vi "CSGaussmeter.init.vi"(0 "i ref in":refnum<vi>, 11 "error in":errorcluster) -> (4 "i ref out":refnum<vi>, 15 "error out":errorcluster)   [LabVIEW 2014, in "CSGaussmeter.lvlib"]
doc: "Dieses VI liest alle Parameter aus dem Gerät aus\n\nThis VI reads all parameters from the device"
uses:
  CSGaussmeter.lvlib
  instr.lib/FH_55/TypeDef/Temp_Unit.ctl
  CS_Core/CSObj/CSObj.lvlib
  CSlibraries/UtilityLib/UtilityLib.lvlib
  CS_Core/CSApplicationBaseClasses/DeviceBase/DeviceBase.lvlib
  instr.lib/FH_55/FH 55.lvlib
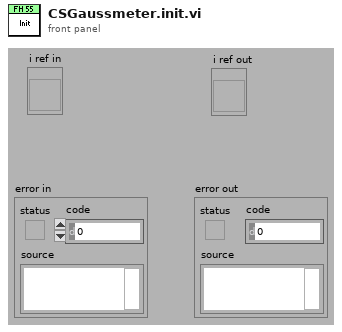
[diagram p1: front panel]
types:
  T1 = typedef "FH 55.lvlib/Temp_Unit.ctl" = enum16{"Temp off", "Celsius", "Fahrenheit"}
  T2 = typedef "CSGaussmeter.lvlib/CSGaussmeter.i attribute.ctl" = cluster{"Name":string, "VISA Resource Name":refnum<visa-resource-name>, "actValues":cluster{" Limit":bool, "Unit ":T3, "Temp_Unit":T1, "Max":T4, " Filter":bool, " Peak":bool, " Auto_Range":bool, "Range":T5, " Rel":bool, " CTemp":bool, " CField":bool, "AC_DC ":bool, "Set_lower":cluster{"Numeric":dbl, "Cancel Button":bool, "Unit":T6}, "Set_upper":cluster{"Numeric":dbl, "Cancel Button":bool, "Unit":T6}, "Set_Rel":cluster{"Numeric":dbl, "Cancel Button":bool, "Unit":T6}, "Zero":bool, " Local":bool, "Reset":bool, " Init":bool}, "FH 55 Gauss-/Teslameter":T7, "MAX_Value":T8, "MIN_Value":T8, "Rel_Value":T8, "Array ":string[], "LIMU":dbl, " LIML":dbl, "Messwerte 2":string, "Messwerte ":cluster{"Numeric":i32, "OK Button":bool}, "serviceID":cluster{"Current ID":i32, "Unit ID":i32, "Temp ID":i32, "Name ID \n":i32, "Visa ID ":i32}, "setValues ":cluster{" Limit":bool, "Unit ":T3, "Temp_Unit":T1, "Max":T4, " Filter":bool, " Peak":bool, " Auto_Range":bool, "Range":T5, " Rel":bool, " CTemp":bool, " CField":bool, "AC_DC ":bool, "Set_lower":cluster{"Numeric":dbl, "Cancel Button":bool, "Unit":T6}, "Set_upper":cluster{"Numeric":dbl, "Cancel Button":bool, "Unit":T6}, "Set_Rel":cluster{"Numeric":dbl, "Cancel Button":bool, "Unit":T6}, "Zero":bool, " Local":bool, "Reset":bool, " Init":bool}}
  T3 = typedef "FH 55.lvlib/Unit.ctl" = enum16{"T", "G", "A/m"}
  T4 = typedef "FH 55.lvlib/Max.ctl" = enum16{"MAX off", "Show MAX", "MAX/MIN"}
  T5 = typedef "FH 55.lvlib/Range.ctl" = enum16{"1", "2", "3", "4", "5", "6", "7"}
  T6 = typedef "FH 55.lvlib/Unit2.ctl" = enum16{"mT", "G", "kA/m"}
  T7 = typedef "FH 55.lvlib/Display.ctl" = cluster{"current value":string, "Limit":string, "Remote":string, "function ":string, "Cluster":cluster{"AC/DC":string, "Auto":string, "Filter":string, "Range":string, "Rel":string, "Peak":string}}
  T8 = typedef "FH 55.lvlib/Value_String.ctl" = cluster{"Numeric":dbl, "String":string}
  T9 = cluster{"VISA Resource Name":refnum<visa-resource-name>}
  T10 = typedef "FH 55.lvlib/VisaCluster.ctl" = cluster{"VISA Resource Name":refnum<visa-resource-name>}
  T11 = cluster{"Numeric":dbl, "Cancel Button":bool, "Unit":T6}
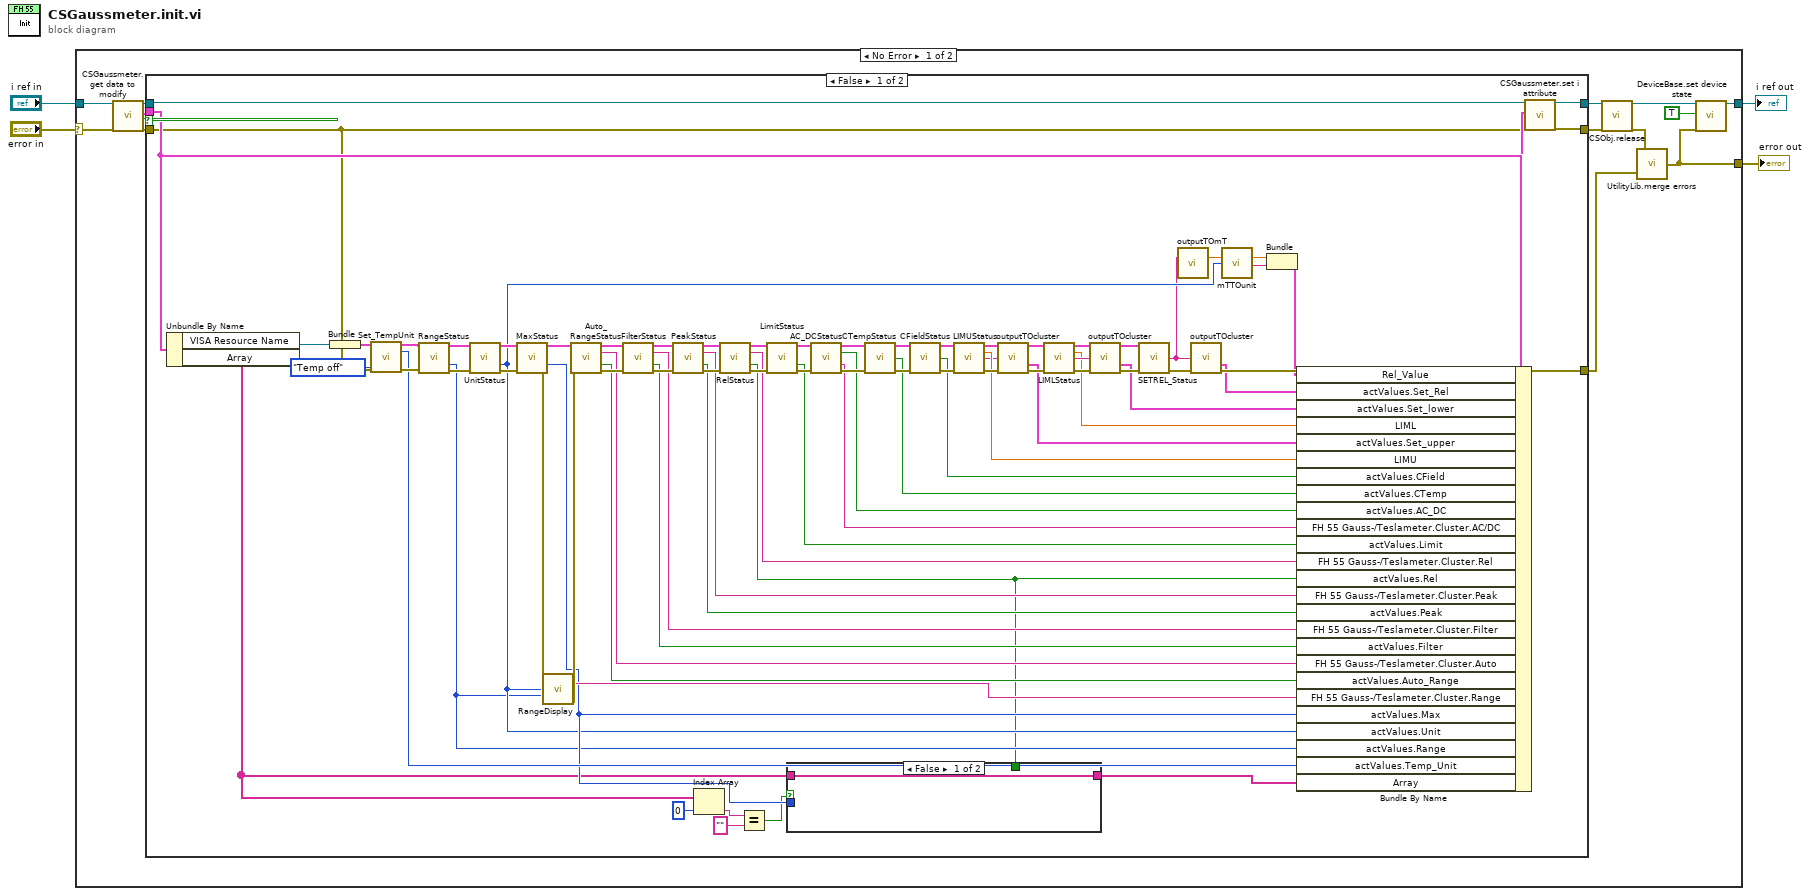
[diagram p0: block diagram]
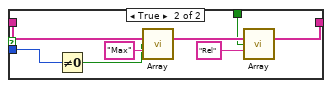
[diagram p2: hidden frame]
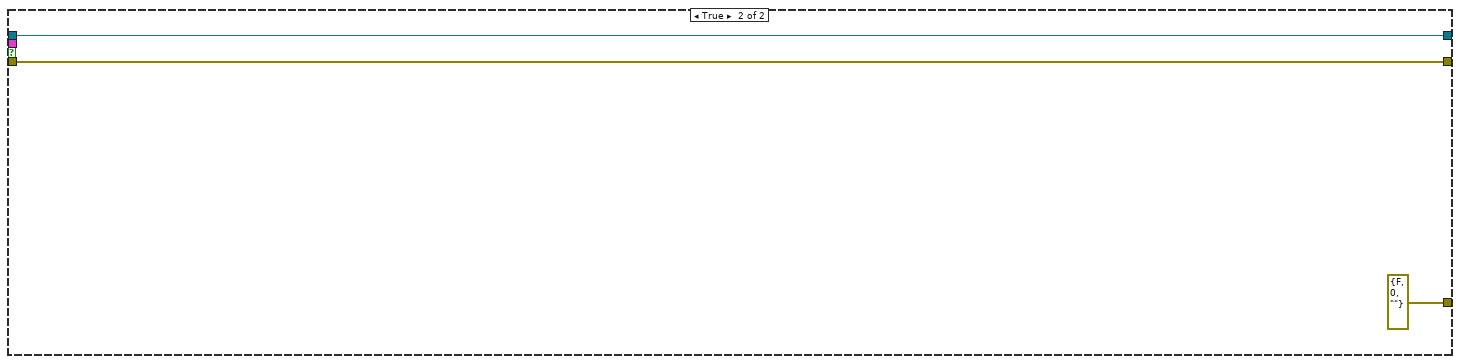
[diagram p3: hidden frame]
diagram:
  n1 = case shown="No Error" "error in" {
    selector: "error in" -> [w9 w109]
    tunnel: "i ref in" -> [w10 w110]
    tunnel: [w12 w110] -> w2
    tunnel: [w11 w109] -> w1
    frame No Error {
      n2 = call "CSGaussmeter.get data to modify.vi"("i ref in"=w10, "error in (no error)"=w9) -> ("i ref out"=w5:refnum<vi>, "i attribute"=w6:T2, "timed out"=w7:bool, "error out"=w8:errorcluster)  [unwired: 14 in]
      n3 = case shown="False" w7 {
        tunnel: w5 -> [w58 w106]
        tunnel: w8 -> [w55 w108]
        tunnel: w6 -> [w63 _]
        tunnel: [w57 w108] -> w17
        tunnel: [w53 errorcluster {"status"=FALSE, "code"=0, "source"=""} ("error out")] -> w18
        tunnel: [w59 w106] -> w15
        frame False {
          n4 = Unbundle By Name(w63) -> ("VISA Resource Name"=w96:refnum<visa-resource-name>, "Array"=w32:string[])
          n5 = Bundle("VISA Resource Name"=w96) -> (w60:T9)  [unwired: 1 in]
          n6 = call "Set_TempUnit.vi"("VisaCluster"=w60, "Temp_Unit"=Temp_Unit."Temp off", "error in (no error)"=w55) -> ("VisaCluster"=w72:T10, "Temp_Unit"=w46:T1, "error out"=w71:errorcluster)  [unwired: 9 in, 1 out]
          n7 = call "RangeStatus.vi"("VisaCluster"=w72, "error in (no error)"=w71) -> ("VisaCluster"=w80:T10, "Range"=w34:T5, "error out"=w78:errorcluster)  [unwired: 10 in, 1 out]
          n8 = call "UnitStatus.vi"("VisaCluster"=w80, "error in (no error)"=w78) -> ("VisaCluster"=w79:T10, "Unit"=w35:T3, "error out"=w77:errorcluster)  [unwired: 10 in, 1 out]
          n9 = call "MaxStatus.vi"("VisaCluster"=w79, "error in (no error)"=w77) -> ("VisaCluster"=w85:T10, "Max"=w36:T4, "error out"=w70:errorcluster)  [unwired: 10 in, 1 out]
          n10 = call "RangeDisplay.vi"("Unit"=w35, "Range"=w34, "error in (no error)"=w70) -> ("Display"=w37:string, "error out"=w69:errorcluster)  [unwired: 10 in, 1 out]
          n11 = call "Auto_RangeStatus.vi"("VisaCluster"=w85, "error in (no error)"=w69) -> ("VisaCluster"=w95:T10, "Display"=w39:string, "Auto_Range"=w38:bool, "error out"=w90:errorcluster)  [unwired: 9 in, 1 out]
          n12 = call "FilterStatus.vi"("VisaCluster"=w95, "error in (no error)"=w90) -> ("VisaCluster"=w94:T10, "Display"=w41:string, "Filter"=w40:bool, "error out"=w89:errorcluster)  [unwired: 9 in, 1 out]
          n13 = call "PeakStatus.vi"("VisaCluster"=w94, "error in (no error)"=w89) -> ("VisaCluster"=w93:T10, "Display"=w43:string, "Peak"=w42:bool, "error out"=w88:errorcluster)  [unwired: 9 in, 1 out]
          n14 = Index Array(array=w32, index=0) -> (element=w30:string)
          n15 = call "RelStatus.vi"("VisaCluster"=w93, "error in (no error)"=w88) -> ("VisaCluster"=w92:T10, "Display"=w44:string, "Rel"=w33:bool, "error out"=w87:errorcluster)  [unwired: 9 in, 1 out]
          n16 = Equal?(x=w30, y="") -> (x = y?=w28:bool)
          n17 = call "LimitStatus.vi"("VisaCluster"=w92, "error in (no error)"=w87) -> ("VisaCluster"=w91:T10, "Limit"=w45:bool, "error out"=w86:errorcluster)  [unwired: 10 in, 1 out]
          n18 = case shown="False" w28 {
            tunnel: [w97 w101] -> w51
            tunnel: w36 -> [_ w100]
            tunnel: w33 -> [_ w99]
            tunnel: w32 -> [w97 w98]
            frame False {
            }
            frame True {
              n19 = Not Equal To 0?(x=w100) -> (x != 0?=w102:bool)
              n20 = call "Array.vi"("Array"=w98, "Boolean"=w102, "String"="Max") -> ("Array"=w103:string[])  [unwired: 12 in]
              n21 = call "Array.vi"("Array"=w103, "Boolean"=w99, "String"="Rel") -> ("Array"=w101:string[])  [unwired: 12 in]
            }
          }
          n22 = call "AC_DCStatus.vi"("VisaCluster"=w91, "error in (no error)"=w86) -> ("VisaCluster"=w84:T10, "AC_DC"=w20:bool, "Display"=w19:string, "error out"=w82:errorcluster)  [unwired: 9 in, 1 out]
          n23 = call "CTempStatus.vi"("VisaCluster"=w84, "error in (no error)"=w82) -> ("VisaCluster"=w83:T10, "CTemp"=w22:bool, "error out"=w81:errorcluster)  [unwired: 10 in, 1 out]
          n24 = call "CFieldStatus.vi"("VisaCluster"=w83, "error in (no error)"=w81) -> ("VisaCluster"=w75:T10, "CField"=w21:bool, "error out"=w76:errorcluster)  [unwired: 10 in, 1 out]
          n25 = call "LIMUStatus.vi"("VisaCluster"=w75, "error in (no error)"=w76) -> ("VisaCluster"=w74:T10, "Numeric"=w27:dbl, "Message Out"=w26:string, "error out"=w68:errorcluster)  [unwired: 10 in]
          n26 = call "outputTOcluster.vi"("Input"=w26, "error in (no error)"=w68) -> ("Set_lower"=w47:T11, "error out"=w67:errorcluster)  [unwired: 11 in, 1 out]
          n27 = call "LIMLStatus.vi"("VisaCluster"=w74, "error in (no error)"=w67) -> ("VisaCluster"=w73:T10, "Numeric"=w24:dbl, "Message Out"=w25:string, "error out"=w66:errorcluster)  [unwired: 10 in]
          n28 = call "outputTOcluster.vi"("Input"=w25, "error in (no error)"=w66) -> ("Set_lower"=w48:T11, "error out"=w65:errorcluster)  [unwired: 11 in, 1 out]
          n29 = call "SETREL_Status.vi"("VisaCluster"=w73, "error in (no error)"=w65) -> ("Answer"=w23:string, "error out"=w54:errorcluster)  [unwired: 10 in, 2 out]
          n30 = call "outputTOmT.vi"("Input"=w23) -> ("Numeric"=w64:dbl)  [unwired: 13 in, 1 out]
          n31 = call "outputTOcluster.vi"("Input"=w23, "error in (no error)"=w54) -> ("Set_lower"=w49:T11, "error out"=w53:errorcluster)  [unwired: 11 in, 1 out]
          n32 = call "mTTOunit.vi"("Numeric"=w64, "Unit"=w35) -> ("Numeric 2"=w62:dbl, "Display"=w61:string)  [unwired: 11 in, 1 out]
          n33 = Bundle("Numeric 2"=w62, "Display"=w61) -> (w50:cluster{"Numeric 2":dbl, "Display":string})  [unwired: 1 in]
          n34 = Bundle By Name(cluster=w63, "Rel_Value"=w50, "actValues.Set_Rel"=w49, "actValues.Set_lower"=w48, "LIML"=w24, "actValues.Set_upper"=w47, "LIMU"=w27, "actValues.CField"=w21, "actValues.CTemp"=w22, "actValues.AC_DC"=w20, "FH 55 Gauss-/Teslameter.Cluster.AC/DC"=w19, "actValues.Limit"=w45, "FH 55 Gauss-/Teslameter.Cluster.Rel"=w44, "actValues.Rel"=w33, "FH 55 Gauss-/Teslameter.Cluster.Peak"=w43, "actValues.Peak"=w42, "FH 55 Gauss-/Teslameter.Cluster.Filter"=w41, "actValues.Filter"=w40, "FH 55 Gauss-/Teslameter.Cluster.Auto"=w39, "actValues.Auto_Range"=w38, "FH 55 Gauss-/Teslameter.Cluster.Range"=w37, "actValues.Max"=w36, "actValues.Unit"=w35, "actValues.Range"=w34, "actValues.Temp_Unit"=w46, "Array"=w51) -> (w56:T2)
          n35 = call "CSGaussmeter.set i attribute.vi"("i ref in"=w58, "i attribute"=w56, "error in (no error)"=w55) -> ("i ref out"=w59:refnum<vi>, "error out"=w57:errorcluster)  [unwired: 15 in]
        }
        frame True {
        }
      }
      n36 = call "CSObj.release.vi"("i ref in"=w15, "error in (no error)"=w17) -> ("i ref out"=w13:refnum<vi>, "error out"=w16:errorcluster)  [unwired: 16 in]
      n37 = call "UtilityLib.merge errors.vi"("error2 (no error)"=w18, "error1 (no error)"=w16) -> ("error out"=w11:errorcluster)
      n38 = call "DeviceBase.set device state.vi"("i ref in"=w13, "implicit"=TRUE, "error in (no error)"=w11) -> ("i ref out"=w12:refnum<vi>)  [unwired: 14 in, 2 out]
    }
    frame Error {
    }
  }
  "i ref out" <- w2
  "error out" <- w1
